vi "Start Async Queue.vi"(6 "Creator":refnum<data-value>, 8 "Creator Alias":string, 9 "Self Alias":string, 10 "Queue of Queue Self":refnum<queue>, 11 "Queue jettl":refnum<class "Queue jettl.lvclass">) -> (0 "error out":errorcluster)   [LabVIEW 2021, in "jettl.lvlib" / "Base Queue jettl.lvlib" / "Base Queue jettl.lvclass"]
uses:
  Base Queue jettl.lvclass
  Queue jettl/Queue jettl.lvclass
  Msg Strategy/Msg Strategy.lvclass
  Actor Queue.vi
  Base Queue jettl.lvclass/Base Queue jettl.ctl
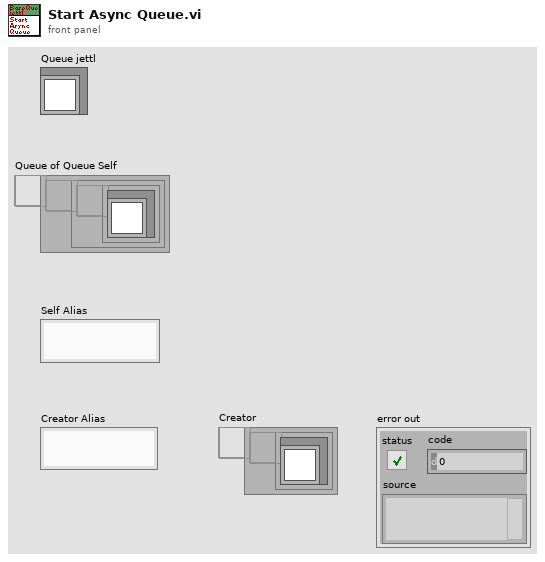
[diagram p1: front panel]
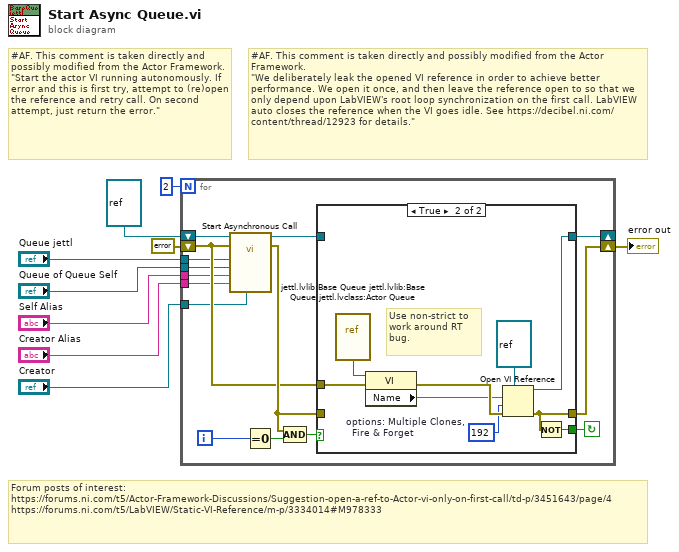
[diagram p0: block diagram]
diagram:
  # "Forum posts of interest:\nhttps://forums.ni.com/t5/Actor-Framework-Discussions/Suggestion-open-a-ref-to-Actor-vi-only-on-first-call/td-p/3451643/page/4\nhttps://forums.ni.com/t5/LabVIEW/Static-VI-Reference/m-p/3334014#M978333"
  # "#AF. This comment is taken directly and possibly modified from the Actor Framework.\n\"We deliberately leak the opened VI reference in order to achieve better performance. We open it once, and then leave the reference open to so that we only depend upon LabVIEW's root loop synchronization on the first call. LabVIEW auto closes the reference when the VI goes idle. See https://decibel.ni.com/content/thread/12923 for details.\""
  # "#AF. This comment is taken directly and possibly modified from the Actor Framework.\n\"Start the actor VI running autonomously. If error and this is first try, attempt to (re)open the reference and retry call. On second attempt, just return the error.\""
  n1 = for {
    N: 2 -> [_]
    shift-right: [w24] -> _
    shift-left: refnum<vi> refnum -> [w23]
    shift-right: [w21] -> w7
    shift-left: errorcluster {"status"=FALSE, "code"=0, "source"=""} ("error out") -> [w15]
    tunnel: "Queue jettl" -> [w14]
    tunnel: "Queue of Queue Self" -> [w13]
    tunnel: "Self Alias" -> [w12]
    tunnel: "Creator Alias" -> [w11]
    tunnel: "Creator" -> [w10]
    i -> [w18]
    stop <- w16 continue-if-true
    n2 = call-by-ref "Start Asynchronous Call"(reference=w23, error in=w15, "Creator"=w10, "Creator Alias"=w11, "Self Alias"=w12, "Queue of Queue Self"=w13, "Queue jettl"=w14) -> (reference out=w22:refnum<vi>, error out=w17:errorcluster)  [unwired: 7 in]
    n3 = Equal To 0?(x=w18) -> (x = 0?=w19:bool)
    n4 = Compound Arithmetic op=AND(w17, w19) -> (w20:bool)
    n5 = case shown="True" w20 {
      tunnel: [w26 w32] -> w24
      tunnel: [w25 w30] -> w21
      tunnel: w22 -> [w26 _]
      tunnel: w17 -> [w25 _]
      tunnel: [_ w31] -> w16
      tunnel: w15 -> [_ w29]
      frame False {
      }
      frame True {
        w33 = 192  # options: Multiple Clones,   Fire & Forget
        # "Use non-strict to work around RT bug."
        n6 = vi-ref "jettl.lvlib:Base Queue jettl.lvlib:Base Queue jettl.lvclass:Actor Queue.vi"() -> (w28:refnum<vi>)
        n7 = property class="VI"(reference=w28, error in=w29) -> (error out=w35:errorcluster, "Name"=w34:string)  [unwired: 1 out]
        n8 = Open VI Reference(type specifier VI Refnum (for type only)=refnum<vi> refnum, vi path=w34, options=w33, error in (no error)=w35) -> (vi reference=w32:refnum<vi>, error out=w30:errorcluster)  [unwired: 2 in]
        n9 = Not(x=w30) -> (.not. x?=w31:bool)
      }
    }
  }
  "error out" <- w7
